vi "CmdExe._Test Simple Exe Run Check.vi"() -> ()   [LabVIEW 2018]
panel:
  out "error out":errorcluster
  in  "Path":path
  out "return code":i32
  out "standard error":string
  out "standard output":string
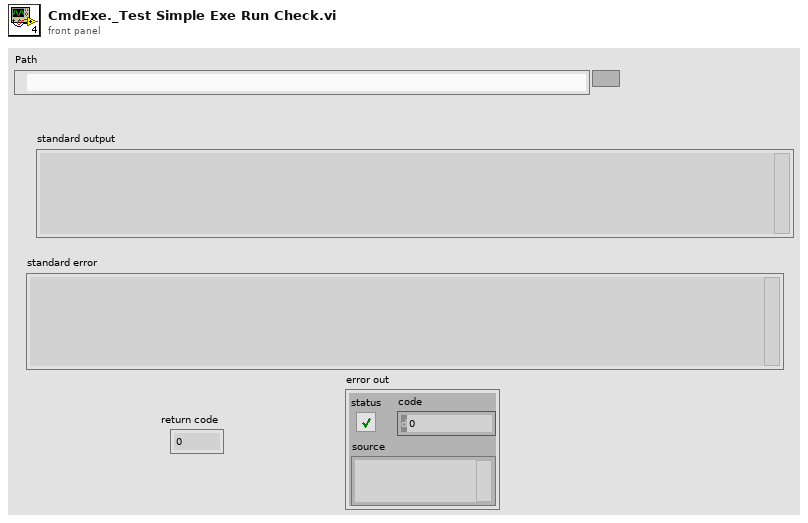
[diagram p1: front panel]
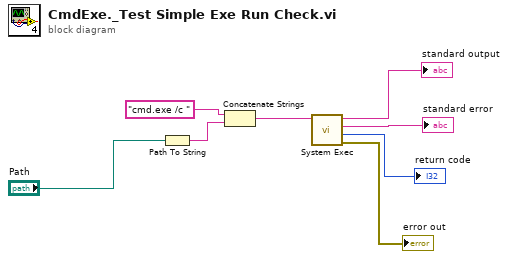
[diagram p0: block diagram]
diagram:
  n1 = Path To String(path="Path") -> (string=w3:string)
  n2 = Concatenate Strings("cmd.exe /c ", w3) -> (w8:string)
  n3 = call <vilib>:"System Exec.vi"("command line"=w8) -> ("error out"=→"error out":errorcluster, "return code"=→"return code":i32, "standard error"=→"standard error":string, "standard output"=→"standard output":string)  [unwired: 7 in]
